vi "Get Status.vi"(8 "Error In":errorcluster) -> (0 "Error Out":errorcluster, 2 "No. Of Elements in Queue":i32, 3 "Queue Name":string)   [LabVIEW 2016, in "Error Manager.lvlib" / "Log To File Loop Queue.lvclass"]
doc: "Returns the queue name and number of elements currently in the queue. Does not remove (dequeue) any element from the queue."
uses:
  Log To File Loop Queue.lvclass
  Queue Reference (library variable).vi
panel:
  # "Input\nInputs to the VI"
  # "Development\nControls or indicators that are useful for development or testing, but which are not outputs of the VI."
  # "Output\nOutputs of the VI"
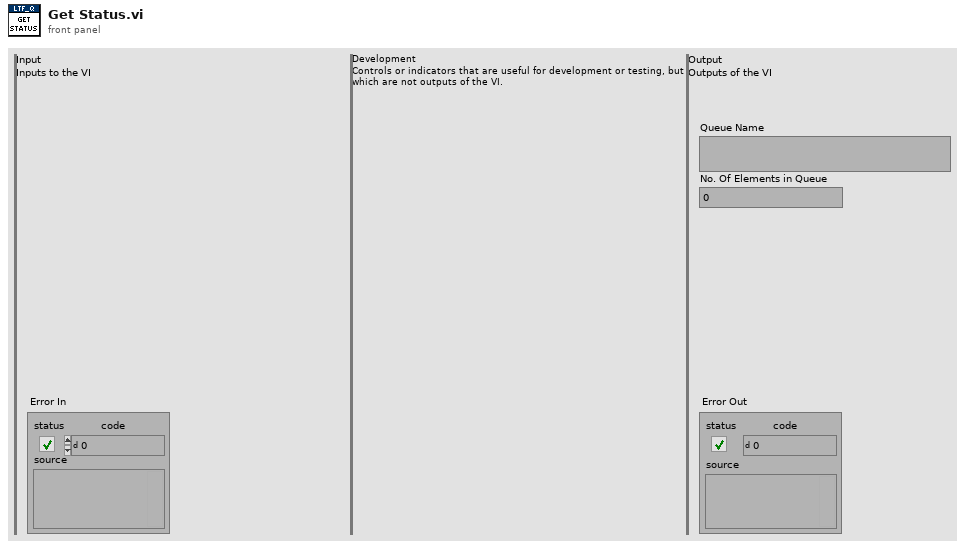
[diagram p1: front panel]
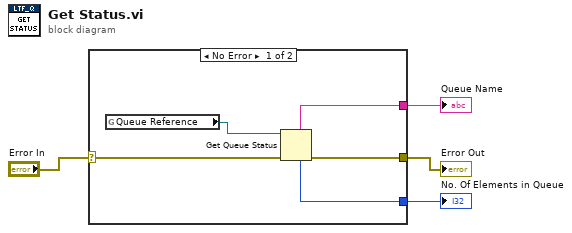
[diagram p0: block diagram]
diagram:
  n1 = case shown="No Error" "Error In" {
    selector: "Error In" -> [w8 w10]
    tunnel: [w9 w10] -> w3
    tunnel: [w7 _] -> w2
    tunnel: [w6 _] -> w1
    frame No Error {
      n2 = global read "Queue Reference (library variable).vi" "Queue Reference"() -> (w5:refnum<queue>)
      n3 = Get Queue Status(queue=w5, error in (no error)=w8) -> (queue name=w6:string, error out=w9:errorcluster, # elements in queue=w7:i32)  [unwired: 1 in, 5 out]
    }
    frame Error {
    }
  }
  "Error Out" <- w3
  "No. Of Elements in Queue" <- w2
  "Queue Name" <- w1
